vi "ConnectCheckReport.vi"(1 "通信状态":bool) -> ()   [LabVIEW 2018]
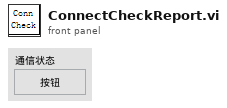
[diagram p1: front panel]
types:
  T1 = cluster{"任务":cluster{"功率任务":bool, "能量任务":bool, "时间波形任务":bool, "光谱任务":bool, "偏振任务":bool, "近远场任务":bool}, "通信":cluster{"功率通信":bool, "能量通信":bool, "时间波形通信":bool, "光谱通信":bool, "偏振通信":bool, "近远场通信":bool}}
  T2 = enum16{"光谱测量", "功率测量", "能量测量", "时间波形", "偏振测量", "近远场"}
  T3 = cluster{"功率通信":bool, "能量通信":bool, "时间波形通信":bool, "光谱通信":bool, "偏振通信":bool, "近远场通信":bool}
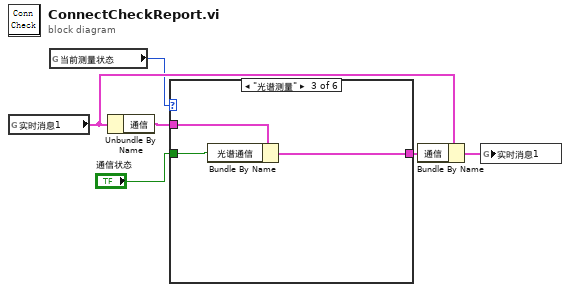
[diagram p0: block diagram]
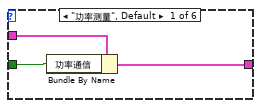
[diagram p2: hidden frame]
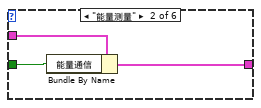
[diagram p3: hidden frame]
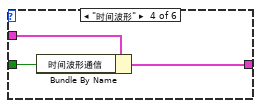
[diagram p4: hidden frame]
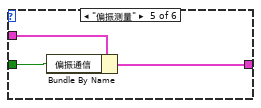
[diagram p5: hidden frame]
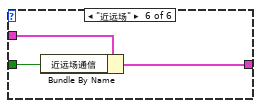
[diagram p6: hidden frame]
diagram:
  n1 = global read "globalMessage.vi" "实时消息1"() -> (w6:T1)
  n2 = global read "参数.vi" "当前测量状态"() -> (w4:T2)
  n3 = Unbundle By Name(w6) -> ("通信"=w3:T3)
  n4 = case shown="\"光谱测量\"" w4 {
    tunnel: w3 -> [w9 w12 w15 w18 w21 w24]
    tunnel: [w8 w11 w14 w17 w20 w23] -> w2
    tunnel: "通信状态" -> [w7 w10 w13 w16 w19 w22]
    frame "功率测量", Default {
      n5 = Bundle By Name(cluster=w9, "功率通信"=w7) -> (w8:T3)
    }
    frame "能量测量" {
      n6 = Bundle By Name(cluster=w12, "能量通信"=w10) -> (w11:T3)
    }
    frame "光谱测量" {
      n7 = Bundle By Name(cluster=w15, "光谱通信"=w13) -> (w14:T3)
    }
    frame "时间波形" {
      n8 = Bundle By Name(cluster=w18, "时间波形通信"=w16) -> (w17:T3)
    }
    frame "偏振测量" {
      n9 = Bundle By Name(cluster=w21, "偏振通信"=w19) -> (w20:T3)
    }
    frame "近远场" {
      n10 = Bundle By Name(cluster=w24, "近远场通信"=w22) -> (w23:T3)
    }
  }
  n11 = Bundle By Name(cluster=w6, "通信"=w2) -> (w5:T1)
  n12 = global write "globalMessage.vi" "实时消息1"(w5) -> ()
